vi "ComputeWfmScalar.vi"(6 "GrpCfg":T1, 7 "Speed":T2, 8 "error in (no error)":errorcluster, 10 "Y Array":sgl[](array[numeric]), 11 "Dynamic in":refnum<class "Dynamic.lvclass">) -> (0 "error out":errorcluster, 2 "Metric":dbl, 3 "Dynamic Out":refnum<class "Dynamic.lvclass">)   [LabVIEW 2012, in "Measurement Channels.lvlib" / "Dynamic.lvclass"]
uses:
  Dynamic.lvclass
  Common/Controls/TE_Designator.ctl
  Common/Controls/Group Timing Info.ctl
  Dynamic.lvclass/Dynamic.ctl
  Class Channel/Read Unit_EU.vi
  <vilib>/Analysis/5stat.llb/RMS (DBL).vi
  <vilib>/Analysis/NI_AALPro.lvlib
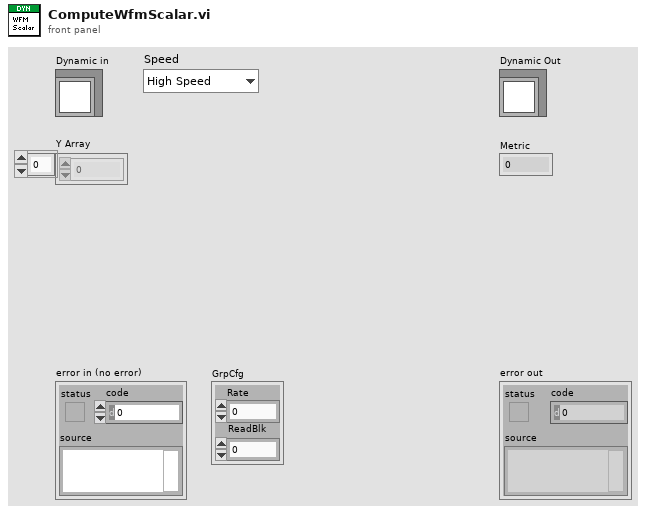
[diagram p1: front panel]
types:
  T1 = typedef "Group Timing Info.ctl" = cluster{"Rate":dbl, "ReadBlk":i32}
  T2 = typedef "TE_Designator.ctl" = enum16{"High Speed", "Low Speed"}
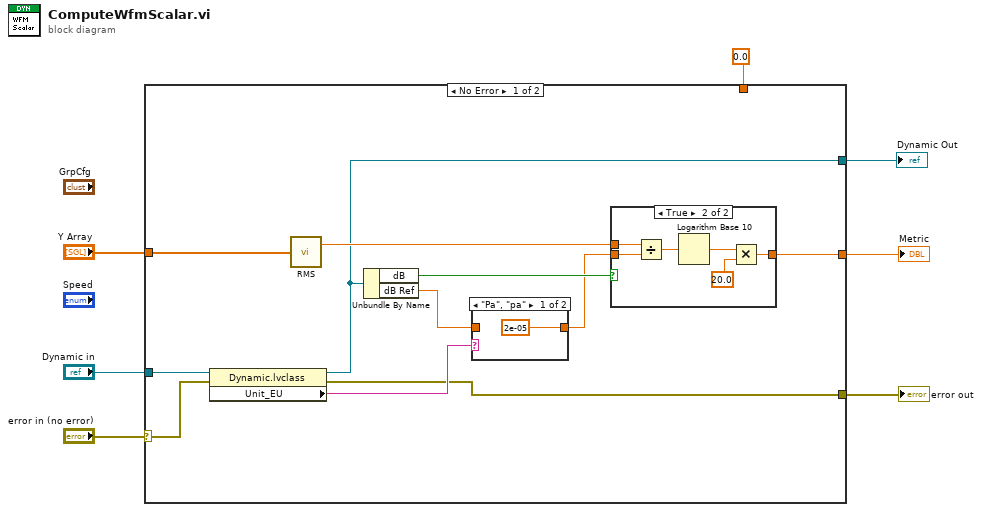
[diagram p0: block diagram]
diagram:
  n1 = case shown="No Error" "error in (no error)" {
    selector: "error in (no error)" -> [w13 w30]
    tunnel: "Dynamic in" -> [w14 w28]
    tunnel: "Y Array" -> [w8 _]
    tunnel: [w9 w30] -> w5
    tunnel: [w10 w29] -> w4
    tunnel: 0.0 ("rms value") -> [_ w29]
    tunnel: [w12 w28] -> w1
    frame No Error {
      n2 = property class="Dynamic.lvclass"(reference=w14, error in=w13) -> (reference out=w12:refnum<class "Dynamic.lvclass">, error out=w9:errorcluster, "Unit_EU"=w11:string)
      n3 = call-poly <vilib>:"RMS.vi"("X"=w8) -> ("rms value"=w18:dbl)  [unwired: 1 out]
      n4 = Unbundle By Name(w12) -> ("dB"=w17:bool, "dB Ref"=w16:dbl)
      n5 = case shown="\"Pa\", \"pa\"" w11 {
        tunnel: w16 -> [_ w20]
        tunnel: [2e-05 ("dB Ref") w20] -> w15
        frame "Pa", "pa" {
        }
        frame Default {
        }
      }
      n6 = case shown="True" w17 {
        tunnel: w18 -> [w21 w27]
        tunnel: w15 -> [_ w26]
        tunnel: [w21 w22] -> w10
        frame False {
        }
        frame True {
          n7 = Divide(x=w27, y=w26) -> (x/y=w25:dbl)
          n8 = Logarithm Base 10(1:w25) -> (0:w24:dbl)
          n9 = Multiply(x=w24, y=20.0 ("x")) -> (x*y=w22:dbl)
        }
      }
    }
    frame Error {
    }
  }
  "error out" <- w5
  "Metric" <- w4
  "Dynamic Out" <- w1
